vi "RTS Door Ops Calculation.vi"(8 "Error In":errorcluster, 11 "Chamber 1-1 in":T1 {"Start Time" format="%<%X\n%x>T"; "End Time" format="%<%X\n%x>T"}) -> (0 "Error Out":errorcluster, 3 "Chamber 1-1 out":T1 {"Start Time" format="%<%X\n%x>T"; "End Time" format="%<%X\n%x>T"})   [LabVIEW 2020]
uses:
  Type Definitions/RTS Door Ops Client.ctl
  Type Definitions/RTS Door Opening Schedule.ctl
  Type Definitions/RTS Door Ops Sequence.ctl
panel:
  out "x-y":dbl
  # "Chamber Conditions:"
  # "Chamber Conditions:"
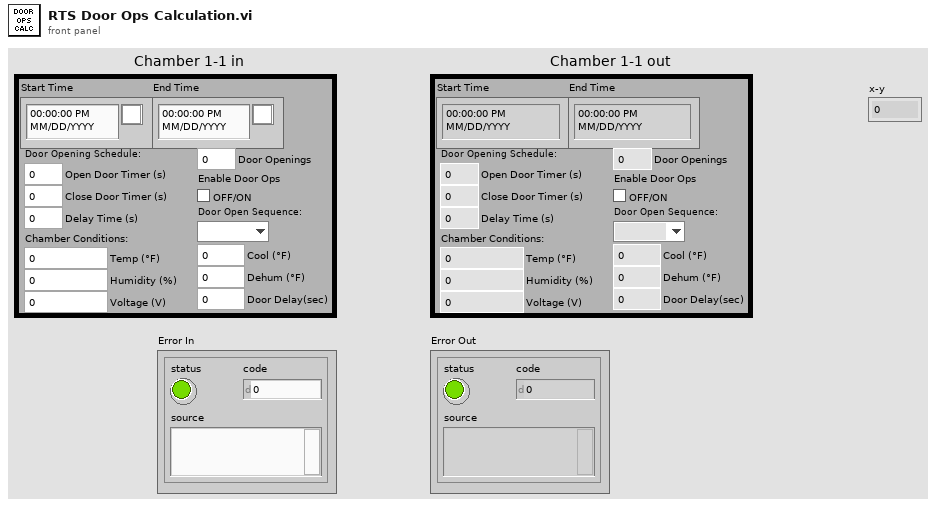
[diagram p1: front panel]
types:
  T1 = typedef "RTS Door Ops Client.ctl" = cluster{"End Time":timestamp, "Start Time":timestamp, "Door Opening Schedule:":T2, "Enable Door Ops":bool, "Door Openings":u32, "Temp (°F)":dbl, "Humidity (%)":dbl, "Voltage (V)":dbl, "Door Open Sequence:":T3, "Door Delay(sec)":dbl, "Dehum (°F)":dbl, "Cool (°F)":dbl}
  T2 = typedef "RTS Door Opening Schedule.ctl" = cluster{"Open Door Timer (s)":dbl, "Delay Time (s)":dbl, "Close Door Timer (s)":dbl}
  T3 = typedef "RTS Door Ops Sequence.ctl" = enum16{"", "1st", "2nd", "3rd"}
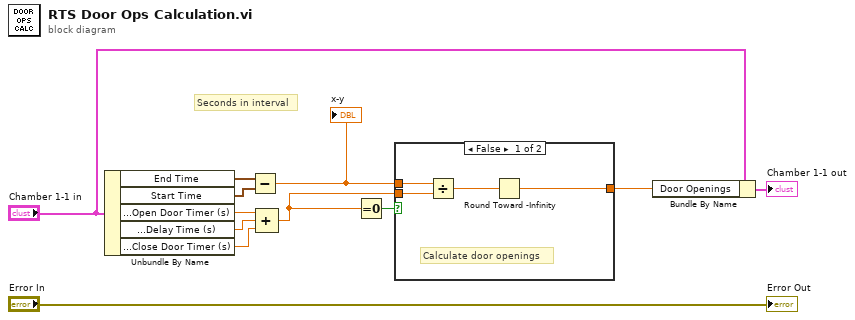
[diagram p0: block diagram]
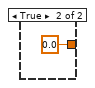
[diagram p2: hidden frame]
diagram:
  # "Seconds in interval"
  n1 = Unbundle By Name("Chamber 1-1 in") -> ("End Time"=w4:timestamp, "Start Time"=w5:timestamp, "Door Opening Schedule:.Open Door Timer (s)"=w6:dbl, "Door Opening Schedule:.Delay Time (s)"=w7:dbl, "Door Opening Schedule:.Close Door Timer (s)"=w8:dbl)
  n2 = Subtract(x=w4, y=w5) -> (x-y=w9:dbl)
  "x-y" <- w9
  n3 = Compound Arithmetic op=ADD(w6, w7, w8) -> (w2:dbl)
  n4 = Equal To 0?(x=w2) -> (x = 0?=w1:bool)
  n5 = case shown="False" w1 {
    tunnel: [w16 0.0] -> w11
    tunnel: w9 -> [w14 _]
    tunnel: w2 -> [w13 _]
    frame False {
      # "Calculate door openings"
      n6 = Divide(x=w14, y=w13) -> (x/y=w15:dbl)
      n7 = Round Toward -Infinity(1:w15) -> (0:w16:dbl)
    }
    frame True {
    }
  }
  n8 = Bundle By Name(cluster="Chamber 1-1 in", "Door Openings"=w11) -> (→"Chamber 1-1 out":T1)
  "Error Out" <- "Error In"
